vi "casetypescraper.vi"() -> ()   [LabVIEW 2025]
uses:
  <extravilib>/ChannelInstances/Event Messenger-c(str,var).lvlib
  Channel Messages/Bundle Module Message/Bundle Module Message.xnode
panel:
  in  "Log Text":string
  in  "Log Button":bool
  out "log":string
  in  "module_interface":map{string, variant}(c390)={"Log"=variant(string ""), "Sum"=variant(cluster{"summand0":dbl, "summand1":dbl} {"summand0"=0.0, "summand1"=0.0})}
  out "error out":errorcluster
  out "x+y":dbl
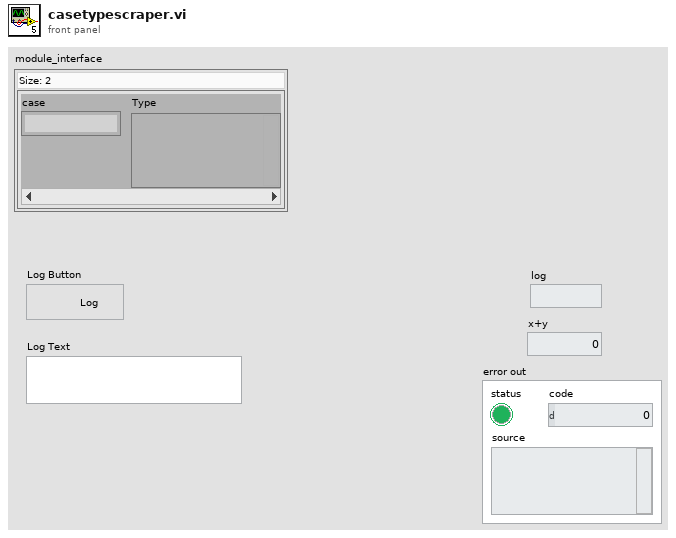
[diagram p1: front panel]
types:
  T1 = typedef "Event Messenger-c(str,var).lvlib/))Channel.ctl" = refnum<queue>
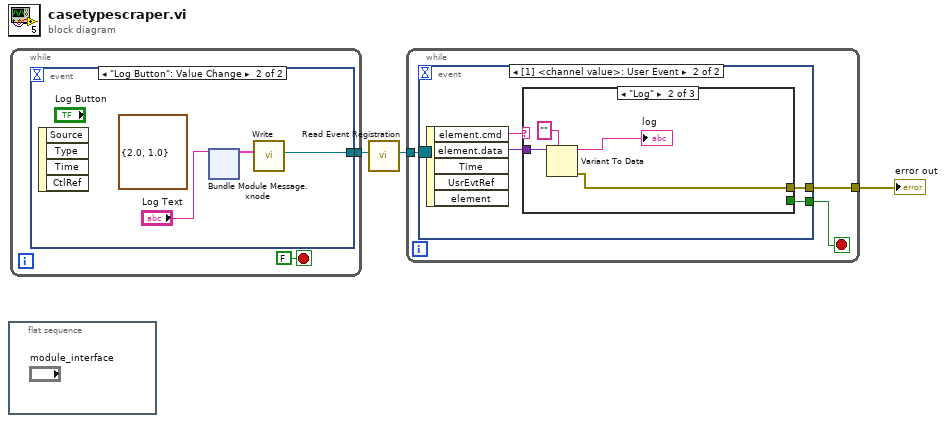
[diagram p0: block diagram]
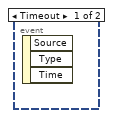
[diagram p2: hidden frame]
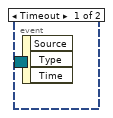
[diagram p3: hidden frame]
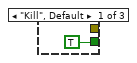
[diagram p4: hidden frame]
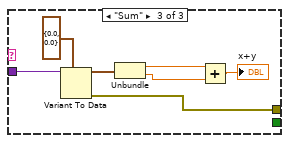
[diagram p5: hidden frame]
diagram:
  n1 = flat-sequence {
    frame #0 {
    }
  }
  n2 = while {
    tunnel: [w5] -> w2
    stop <- FALSE stop-if-true
    n3 = event shown="[1] \"Log Button\": Value Change" {
      selector: _ -> [_ _]
      dyn-events: _ -> [_ _]
      timeout: _ -> [_ _]
      tunnel: [_ w8] -> w5
      event Timeout {
        n4 = event-data() -> ()  [unwired: 1 in, 3 out]
      }
      event "Log Button": Value Change {
        (unwired) cluster{"summand0":dbl, "summand1":dbl} {"summand0"=2.0, "summand1"=1.0} ("data")
        n5 = event-data() -> ()  [unwired: 1 in, 4 out]
        n6 = xnode "Bundle Module Message.xnode"("data"="Log Text") -> ("message"=w7:cluster{"cmd":string, "data":variant})
        n7 = call <extravilib>:"Write.vi"("element"=w7) -> ("channel"=w8:T1)  [unwired: 9 in, 1 out]
      }
    }
  }
  n8 = call <extravilib>:"Read Event Registration.vi"("channel"=w2) -> ("event registration refnum"=w1:refnum<event-registration>)  [unwired: 10 in]
  n9 = while {
    tunnel: w1 -> [w15]
    tunnel: [w14] -> w3
    stop <- w13 stop-if-true
    n10 = event shown="[1] <channel value>: User Event" {
      selector: w15 -> [_ _]
      dyn-events: _ -> [_ _]
      timeout: _ -> [_ _]
      tunnel: [_ w19] -> w14
      tunnel: [_ w16] -> w13
      event Timeout {
        n11 = event-data() -> ()  [unwired: 1 in, 3 out]
      }
      event User Event {
        n12 = event-data() -> ("element.cmd"=w18:string, "element.data"=w17:variant)  [unwired: 1 in, 3 out]
        n13 = case shown="\"Log\"" w18 {
          tunnel: w17 -> [_ w22 w31]
          tunnel: [_ w21 w25] -> w19
          tunnel: [TRUE _ _] -> w16
          frame "Kill", Default {
          }
          frame "Log" {
            n14 = Variant To Data(type="", Variant=w22) -> (data=→"log":string, error out=w21:errorcluster)  [unwired: 1 in]
          }
          frame "Sum" {
            n15 = Variant To Data(type=cluster{"summand0":dbl, "summand1":dbl} {"summand0"=0.0, "summand1"=0.0} ("summands"), Variant=w31) -> (data=w29:cluster{"summand0":dbl, "summand1":dbl}, error out=w25:errorcluster)  [unwired: 1 in]
            n16 = Unbundle(w29) -> ("summand0"=w28:dbl, "summand1"=w27:dbl)
            n17 = Add(x=w28, y=w27) -> (x+y=→"x+y":dbl)
          }
        }
      }
    }
  }
  "error out" <- w3
